vi "pco.camera_SaveMean_Example_IMAQ.vi"() -> ()   [LabVIEW 2019]
uses:
  pco.camera/Camera.lvclass
panel:
  out "rawImage":u16[][](array[numeric])
  out "Image":T1(plugin-control)
  in  "data_format":T2(ring)=enum."Mono16"
  in  "Image Index":u32 max=99
  in  "saveImages":bool
  in  "SavePath":path
  out "Recorded Images":u32
  in  "Quit":bool
  in  "roiY1":u64=2 min=2 max=1040 step=1
  in  "roiX1":u64=2 min=2 max=1392 step=1
  in  "roiY0":u64=1 min=1 max=1039 step=1
  in  "roiX0":u64=1 min=1 max=1391 step=1
  out "Image Height":u16
  out "Image Width":u16
  in  "dwImgCount":u32=10 caption="Required Number of Images" max=4023
  out "Error":errorcluster {"code" format="%x"}
  # "This example shows how to record an image sequence, get the mean of that sequence and save it to file afterwards.\nIt is a good starting point for writing own applications.\nBut it will not be fail save, i.e. doesnt react on errors, just handles them forward to the end\n\nUsage:\nSelect your required image count you want to average over before you start the program.\nOnce started, the camera class will be initialized and images will be recorded automatically.\nTWhen acquisition has finished the mean image is read and shown.\nNow you can crop the image using the ROI parameters and select a file path.\nBy clicking save, the mean image is saved with the selected file format using the current roi setting\nThis also finishes the program and will force an exit of the camera class"
  # "pco.labview"
  # "Camera Setup"
  # "Recording Control"
  # "Parameters for image readout"
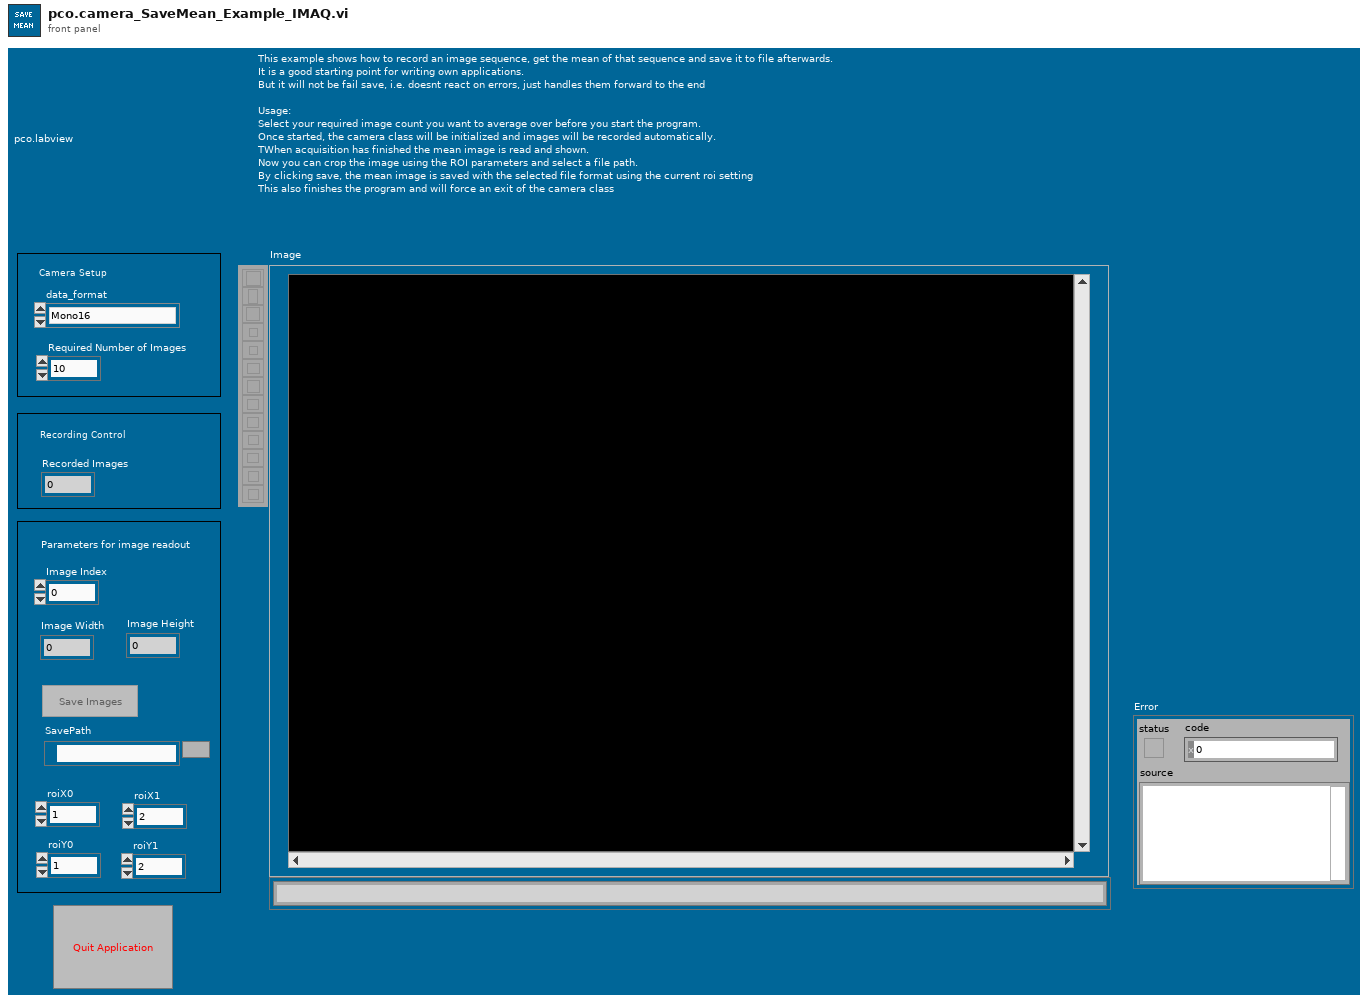
[diagram p1: front panel]
types:
  T1 = typedef "IMAQ Image.ctl" = refnum<image>
  T2 = enum16{"Undefined", "Mono8", "Mono16", "BGRA8", "RGBA8", "BGRA16", "RGBA16", "CompressedMono8"}
  T3 = enum8{"Enabled", "Disabled", "Disabled and Grayed Out"}
  T4 = enum16{"sequence", "sequence non blocking", "ring buffer", "fifo", "sequence_dpcore", "sequence_non_blocking_dpcore", "ring_buffer_dpcore", "fifo_dpcore", "tif", "multitif", "pcoraw", "b16", "dicom", "multidicom"}
  T5 = typedef "Image Type" = u32
  T6 = typedef "Camera.lvclass/binning.ctl" = cluster{"vert":u16, "horz":u16}
  T7 = cluster{"exposure_time_s":dbl, "delay_time_s":dbl, "roi":cluster{"x0":u64, "y0":u64, "x1":u64, "y1":u64}, "timestamp_mode":u16, "pixelrate":u32, "trigger_mode":u16, "acquire_mode":u16, "metadata_mode":u16, "noisefilter_mode":u16, "binning":T6}
  T8 = typedef "Color (U64)" = cluster{"Plane 3 (Blue)":u16, "Plane 2 (Green)":u16, "Plane 1 (Red)":u16, "Plane 4 (alpha)":u16}
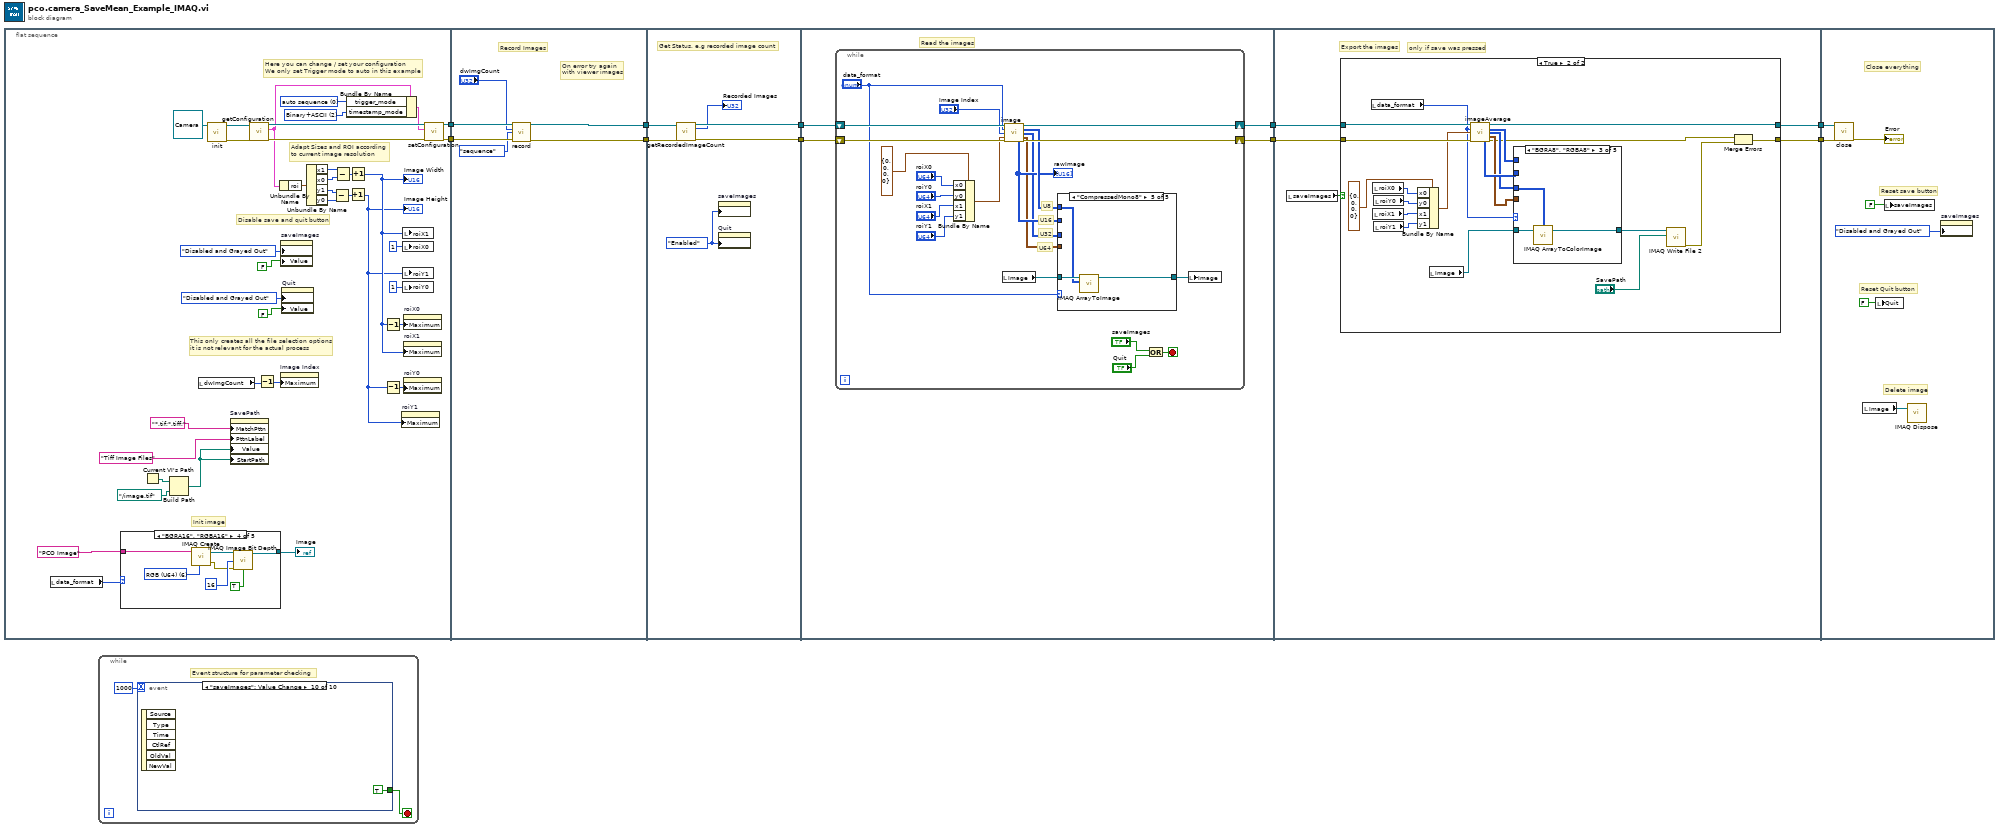
[diagram p0: block diagram]
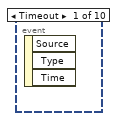
[diagram p2: hidden frame]
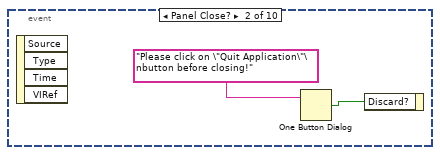
[diagram p3: hidden frame]
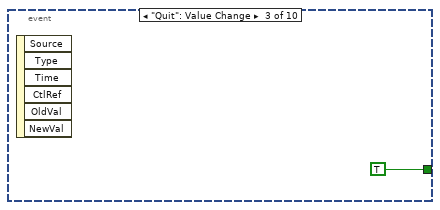
[diagram p4: hidden frame]
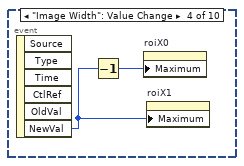
[diagram p5: hidden frame]
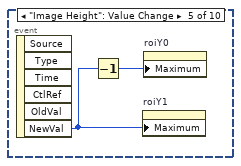
[diagram p6: hidden frame]
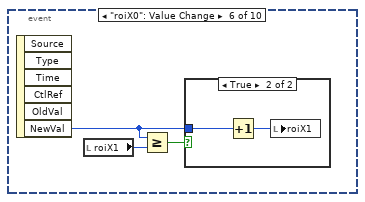
[diagram p7: hidden frame]
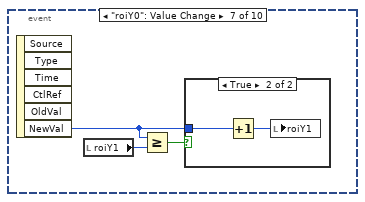
[diagram p9: hidden frame]
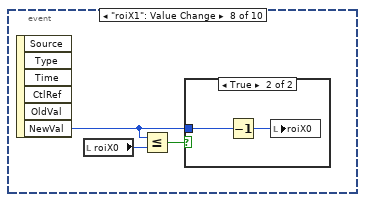
[diagram p11: hidden frame]
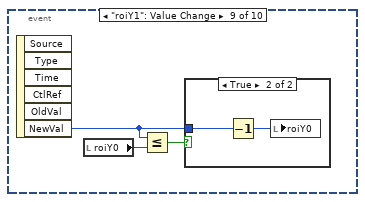
[diagram p13: hidden frame]
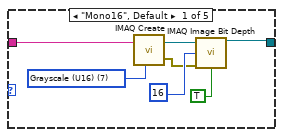
[diagram p15: hidden frame]
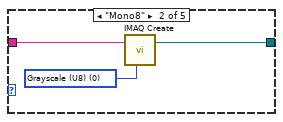
[diagram p16: hidden frame]
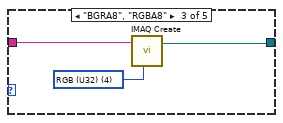
[diagram p17: hidden frame]
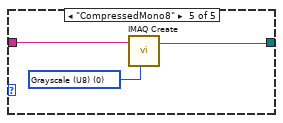
[diagram p18: hidden frame]
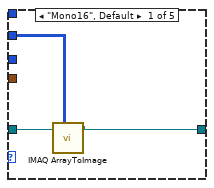
[diagram p19: hidden frame]
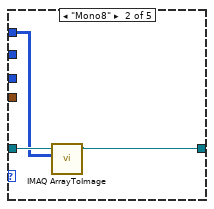
[diagram p20: hidden frame]
diagram:
  n1 = flat-sequence {
    tunnel: [w39] -> w10
    tunnel: [w38] -> w9
    tunnel: w10 -> [w77]
    tunnel: w9 -> [w76]
    tunnel: [w74] -> w8
    tunnel: [w73] -> w7
    tunnel: w8 -> [w83]
    tunnel: w7 -> [w82]
    tunnel: [w81] -> w6
    tunnel: [w80] -> w5
    tunnel: w6 -> [w86]
    tunnel: w5 -> [w87]
    tunnel: [w85] -> w4
    tunnel: [w84] -> w2
    tunnel: w4 -> [w127]
    tunnel: [w126] -> w3
    tunnel: w2 -> [w125]
    tunnel: [w124] -> w1
    tunnel: w3 -> [w172]
    tunnel: w1 -> [w171]
    frame #0 {
      w23 = u16 2 items=["OFF", "Binary", "Binary+ASCII", "ASCII"] ("TimestampMode")
      w45 = u16 0 items=["auto sequence"=0, "software trigger"=1, "external exposure start & software trigger"=2, "external exposure control"=3, "external synchronized"=4, "fast external exposure control"=5, "external CDS control"=6, "slow external exposure control"=7, "external synchronized HDSDI"=258] ("TriggerMode")
      # "Init image"
      # "This only creates all the file selection options\nit is not relevant for the actual process"
      # "Adapt Sizes and ROI according\nto current image resolution"
      # "Disable save and quit button"
      # "Here you can change / set your configuration\nWe only set Trigger mode to auto in this example"
      n2 = local read "data_format"() -> (w13:T2)
      n3 = case shown="\"BGRA16\", \"RGBA16\"" w13 {
        tunnel: "PCO Image" ("Image Name") -> [w54 w58 w60 w67 w70]
        tunnel: [w49 w56 w59 w63 w69] -> w12
        frame "Mono16", Default {
          w55 = T5 7 items=["Grayscale (U8)", "Grayscale (I16)", "Grayscale (SGL)", "Complex (CSG)", "RGB (U32)", "HSL (U32)", "RGB (U64)", "Grayscale (U16)"] ("Image Type")
          n4 = call "IMAQ Create"("Image Name"=w54, "Image Type"=w55) -> ("New Image"=w51:T1, "error out"=w50:errorcluster)  [unwired: 3 in]
          n5 = call "IMAQ Image Bit Depth"("Image"=w51, "Bit Depth (0)"=u32 16, "error in (no error)"=w50, "Get/Set Bit Depth? (Set)"=TRUE) -> ("Image Out"=w49:T1)  [unwired: 9 in, 2 out]
        }
        frame "Mono8" {
          w57 = T5 0 items=["Grayscale (U8)", "Grayscale (I16)", "Grayscale (SGL)", "Complex (CSG)", "RGB (U32)", "HSL (U32)", "RGB (U64)", "Grayscale (U16)"] ("Image Type")
          n6 = call "IMAQ Create"("Image Name"=w58, "Image Type"=w57) -> ("New Image"=w56:T1)  [unwired: 3 in, 1 out]
        }
        frame "BGRA8", "RGBA8" {
          w61 = T5 4 items=["Grayscale (U8)", "Grayscale (I16)", "Grayscale (SGL)", "Complex (CSG)", "RGB (U32)", "HSL (U32)", "RGB (U64)", "Grayscale (U16)"] ("Image Type")
          n7 = call "IMAQ Create"("Image Name"=w60, "Image Type"=w61) -> ("New Image"=w59:T1)  [unwired: 3 in, 1 out]
        }
        frame "BGRA16", "RGBA16" {
          w68 = T5 6 items=["Grayscale (U8)", "Grayscale (I16)", "Grayscale (SGL)", "Complex (CSG)", "RGB (U32)", "HSL (U32)", "RGB (U64)", "Grayscale (U16)"] ("Image Type")
          n8 = call "IMAQ Create"("Image Name"=w67, "Image Type"=w68) -> ("New Image"=w64:T1, "error out"=w62:errorcluster)  [unwired: 3 in]
          n9 = call "IMAQ Image Bit Depth"("Image"=w64, "Bit Depth (0)"=u32 16, "error in (no error)"=w62, "Get/Set Bit Depth? (Set)"=TRUE) -> ("Image Out"=w63:T1)  [unwired: 9 in, 2 out]
        }
        frame "CompressedMono8" {
          w71 = T5 0 items=["Grayscale (U8)", "Grayscale (I16)", "Grayscale (SGL)", "Complex (CSG)", "RGB (U32)", "HSL (U32)", "RGB (U64)", "Grayscale (U16)"] ("Image Type")
          n10 = call "IMAQ Create"("Image Name"=w70, "Image Type"=w71) -> ("New Image"=w69:T1)  [unwired: 3 in, 1 out]
        }
      }
      "Image" <- w12
      n11 = Current VI's Path() -> (path=w20:path)
      n12 = Build Path(base path=w20, name or relative path=path "../image.tif" ("SavePath")) -> (appended path=w17:path)
      n13 = local read "dwImgCount"() -> (w15:u32)
      n14 = call-dynamic "init.vi"("Camera in"=refnum<class "Camera.lvclass"> refnum ("PCOCamera in")) -> ("Camera out"=w47:refnum<class "Camera.lvclass">, "error out"=w46:errorcluster)  [unwired: 8 in]
      n15 = property on="SavePath" class="Path"("MatchPttn"="*.tif;*.tiff;" ("pattern (all files)"), "PttnLabel"="Tiff Image Files" ("pattern label"), "Value"=w17, "StartPath"=w17) -> ()  [unwired: 2 in, 2 out]
      n16 = call-dynamic "getConfiguration.vi"("error in (no error)"=w46, "Camera in"=w47) -> ("error out"=w43:errorcluster, "configuration"=w33:T7, "Camera out"=w44:refnum<class "Camera.lvclass">)  [unwired: 7 in]
      n17 = Decrement(x=w15) -> (x-1=w16:u32)
      n18 = Unbundle By Name(w33) -> ("roi"=w32:cluster{"x0":u64, "y0":u64, "x1":u64, "y1":u64})
      n19 = property on="Image Index" class="DigNum (strict)"("Maximum"=w16) -> ()  [unwired: 2 in, 2 out]
      n20 = property on="saveImages" class="Bool (strict)"("DisabledEnum"=T3."Disabled and Grayed Out" ("Disabled"), "Value"=FALSE ("Stop")) -> ()  [unwired: 2 in, 2 out]
      n21 = property on="Quit" class="Bool (strict)"("DisabledEnum"=T3."Disabled and Grayed Out" ("Disabled"), "Value"=FALSE ("Stop")) -> ()  [unwired: 2 in, 2 out]
      n22 = Unbundle By Name(w32) -> ("x1"=w30:u64, "x0"=w31:u64, "y1"=w28:u64, "y0"=w29:u64)
      n23 = Subtract(x=w28, y=w29) -> (x-y=w26:u64)
      n24 = Subtract(x=w30, y=w31) -> (x-y=w27:u64)
      n25 = Bundle By Name(cluster=w33, "trigger_mode"=w45, "timestamp_mode"=w23) -> (w42:T7)
      n26 = Increment(x=w26) -> (x+1=w24:u64)
      "Image Height" <- w24
      n27 = Increment(x=w27) -> (x+1=w25:u64)
      "Image Width" <- w25
      n28 = Decrement(x=w25) -> (x-1=w35:u64)
      n29 = Decrement(x=w24) -> (x-1=w34:u64)
      n30 = property on="roiY1" class="DigNum (strict)"("Maximum"=w24) -> ()  [unwired: 2 in, 2 out]
      n31 = local write "roiX1"(w25) -> ()
      n32 = local write "roiX0"(u16 1 ("roiY0")) -> ()
      n33 = local write "roiY1"(w24) -> ()
      n34 = local write "roiY0"(u16 1 ("roiY0")) -> ()
      n35 = property on="roiX0" class="DigNum (strict)"("Maximum"=w35) -> ()  [unwired: 2 in, 2 out]
      n36 = property on="roiX1" class="DigNum (strict)"("Maximum"=w25) -> ()  [unwired: 2 in, 2 out]
      n37 = property on="roiY0" class="DigNum (strict)"("Maximum"=w34) -> ()  [unwired: 2 in, 2 out]
      n38 = call-dynamic "setConfiguration.vi"("error in (no error)"=w43, "configuration"=w42, "Camera in"=w44) -> ("error out"=w38:errorcluster, "Camera out"=w39:refnum<class "Camera.lvclass">)  [unwired: 7 in]
    }
    frame #1 {
      # "On error try again \nwith viewer images"
      # "Record Images"
      n39 = call-dynamic "record.vi"("Camera in"=w77, "num_images"="dwImgCount", "record_mode"=T4."sequence", "error in (no error)"=w76) -> ("Camera out"=w74:refnum<class "Camera.lvclass">, "error out"=w73:errorcluster)  [unwired: 10 in]
    }
    frame #2 {
      w78 = T3."Enabled" ("Disabled")
      # "Get Status, e.g recorded image count"
      n40 = call-dynamic "getRecordedImageCount.vi"("Camera in"=w83, "error in (no error)"=w82) -> ("Camera out"=w81:refnum<class "Camera.lvclass">, "recorded_image_count"=→"Recorded Images":u32, "error out"=w80:errorcluster)  [unwired: 11 in]
      n41 = property on="saveImages" class="Bool (strict)"("DisabledEnum"=w78) -> ()  [unwired: 2 in, 2 out]
      n42 = property on="Quit" class="Bool (strict)"("DisabledEnum"=w78) -> ()  [unwired: 2 in, 2 out]
    }
    frame #3 {
      # "Read the images"
      n43 = while {
        shift-right: [w106] -> w85
        shift-left: w86 -> [w108]
        shift-right: [w101] -> w84
        shift-left: w87 -> [w107]
        stop <- w99 stop-if-true
        # "U64"
        # "U32"
        # "U16"
        # "U8"
        n44 = Bundle By Name(cluster=cluster{"x0":u64, "y0":u64, "x1":u64, "y1":u64} {"x0"=0, "y0"=0, "x1"=0, "y1"=0} ("roi"), "x0"="roiX0", "y0"="roiY0", "x1"="roiX1", "y1"="roiY1") -> (w97:cluster{"x0":u64, "y0":u64, "x1":u64, "y1":u64})
        n45 = local read "Image"() -> (w90:T1)
        n46 = call-dynamic "image.vi"("Camera in"=w108, "data_format"="data_format", "image_index"="Image Index", "roi"=w97, "error in (no error)"=w107) -> ("Camera out"=w106:refnum<class "Camera.lvclass">, "image (U8)"=w94:u8[][], "image (U32)"=w92:u32[][], "image (U64)"=w91:T8[][], "raw_image (U16)"=w93:u16[][], "error out"=w101:errorcluster)  [unwired: 3 in, 2 out]
        "rawImage" <- w93
        n47 = case shown="\"CompressedMono8\"" "data_format" {
          tunnel: w90 -> [w111 w114 w117 w120 w123]
          tunnel: [w109 w112 w116 w118 w122] -> w89
          tunnel: w91 -> [_ _ _ w119 _]
          tunnel: w92 -> [_ _ w115 _ _]
          tunnel: w94 -> [_ w113 _ _ w121]
          tunnel: w93 -> [w110 _ _ _ _]
          frame "Mono16", Default {
            n48 = call "IMAQ ArrayToImage"("Image Pixels (U16)"=w110, "Image"=w111) -> ("Image Out"=w109:T1)  [unwired: 8 in, 1 out]
          }
          frame "Mono8" {
            n49 = call "IMAQ ArrayToImage"("Image Pixels (U8)"=w113, "Image"=w114) -> ("Image Out"=w112:T1)  [unwired: 8 in, 1 out]
          }
          frame "BGRA8", "RGBA8" {
            n50 = call "IMAQ ArrayToColorImage"("Image Pixels (U32)"=w115, "Image"=w117) -> ("Image Out"=w116:T1)  [unwired: 3 in, 1 out]
          }
          frame "BGRA16", "RGBA16" {
            n51 = call "IMAQ ArrayToColorImage"("Image"=w120, "Image Pixels (U64)"=w119) -> ("Image Out"=w118:T1)  [unwired: 3 in, 1 out]
          }
          frame "CompressedMono8" {
            n52 = call "IMAQ ArrayToImage"("Image Pixels (U8)"=w121, "Image"=w123) -> ("Image Out"=w122:T1)  [unwired: 8 in, 1 out]
          }
        }
        n53 = Or(x="saveImages", y="Quit") -> (x .or. y?=w99:bool)
        n54 = local write "Image"(w89) -> ()
      }
    }
    frame #4 {
      # "only if save was pressed"
      # "Export the images"
      n55 = local read "saveImages"() -> (w128:bool)
      n56 = case shown="True" w128 {
        tunnel: w127 -> [w130 w149]
        tunnel: [w130 w138] -> w126
        tunnel: w125 -> [w129 w150]
        tunnel: [w129 w136] -> w124
        frame False {
        }
        frame True {
          n57 = local read "data_format"() -> (w134:T2)
          n58 = local read "roiX0"() -> (w147:u64)
          n59 = local read "roiX1"() -> (w145:u64)
          n60 = local read "roiY0"() -> (w146:u64)
          n61 = local read "roiY1"() -> (w144:u64)
          n62 = Bundle By Name(cluster=cluster{"x0":u64, "y0":u64, "x1":u64, "y1":u64} {"x0"=0, "y0"=0, "x1"=0, "y1"=0} ("roi"), "x0"=w147, "y0"=w146, "x1"=w145, "y1"=w144) -> (w143:cluster{"x0":u64, "y0":u64, "x1":u64, "y1":u64})
          n63 = local read "Image"() -> (w135:T1)
          n64 = call-dynamic "imageAverage.vi"("Camera in"=w149, "data_format"=w134, "roi"=w143, "error in (no error)"=w150) -> ("Camera out"=w138:refnum<class "Camera.lvclass">, "image (U8)"=w142:u8[][], "image (U32)"=w140:u32[][], "image (U64)"=w139:T8[][], "raw_image (U16)"=w141:u16[][], "error out"=w137:errorcluster)  [unwired: 6 in]
          n65 = case shown="\"BGRA8\", \"RGBA8\"" w134 {
            tunnel: w135 -> [w153 w156 w159 w162 w165]
            tunnel: [w151 w154 w158 w160 w164] -> w132
            tunnel: w139 -> [_ _ _ w161 _]
            tunnel: w140 -> [_ _ w157 _ _]
            tunnel: w142 -> [_ w155 _ _ w163]
            tunnel: w141 -> [w152 _ _ _ _]
            frame "Mono16", Default {
              n66 = call "IMAQ ArrayToImage"("Image Pixels (U16)"=w152, "Image"=w153) -> ("Image Out"=w151:T1)  [unwired: 8 in, 1 out]
            }
            frame "Mono8" {
              n67 = call "IMAQ ArrayToImage"("Image Pixels (U8)"=w155, "Image"=w156) -> ("Image Out"=w154:T1)  [unwired: 8 in, 1 out]
            }
            frame "BGRA8", "RGBA8" {
              n68 = call "IMAQ ArrayToColorImage"("Image Pixels (U32)"=w157, "Image"=w159) -> ("Image Out"=w158:T1)  [unwired: 3 in, 1 out]
            }
            frame "BGRA16", "RGBA16" {
              n69 = call "IMAQ ArrayToColorImage"("Image"=w162, "Image Pixels (U64)"=w161) -> ("Image Out"=w160:T1)  [unwired: 3 in, 1 out]
            }
            frame "CompressedMono8" {
              n70 = call "IMAQ ArrayToImage"("Image Pixels (U8)"=w163, "Image"=w165) -> ("Image Out"=w164:T1)  [unwired: 8 in, 1 out]
            }
          }
          n71 = call-poly "IMAQ Write File 2"("File Path"="SavePath", "Image"=w132) -> ("error out"=w133:errorcluster)  [unwired: 8 in, 1 out]
          n72 = Merge Errors(w137, w133) -> (w136:errorcluster)
        }
      }
    }
    frame #5 {
      # "Delete image"
      # "Reset Quit button"
      # "Close everything"
      # "Reset save button"
      n73 = call-dynamic "close.vi"("error in (no error)"=w171, "Camera in"=w172) -> ("error out"=→"Error":errorcluster)  [unwired: 9 in]
      n74 = local read "Image"() -> (w166:T1)
      n75 = local write "Quit"(FALSE ("Stop")) -> ()
      n76 = local write "saveImages"(FALSE ("Stop")) -> ()
      n77 = call "IMAQ Dispose"("Image"=w166) -> ()  [unwired: 5 in, 1 out]
      n78 = property on="saveImages" class="Bool (strict)"("DisabledEnum"=T3."Disabled and Grayed Out" ("Disabled")) -> ()  [unwired: 2 in, 2 out]
    }
  }
  n79 = while {
    stop <- w173 stop-if-true
    # "Event structure for parameter checking"
    n80 = event shown="[9] \"saveImages\": Value Change" {
      selector: _ -> [_ _ _ _ _ _ _ _ _ _]
      dyn-events: _ -> [_ _ _ _ _ _ _ _ _ _]
      timeout: 1000 -> [_ _ _ _ _ _ _ _ _ _]
      tunnel: [_ _ TRUE _ _ _ _ _ _ TRUE] -> w173
      event Timeout {
        n81 = event-data() -> ()  [unwired: 1 in, 3 out]
      }
      event Panel Close? {
        n82 = event-data() -> ()  [unwired: 1 in, 4 out]
        n83 = One Button Dialog(message="Please click on \"Quit Application\"\nbutton before closing!") -> (true=w175:bool)  [unwired: 1 in]
        n84 = event-data("Discard?"=w175) -> ()  [unwired: 1 in, 1 out]
      }
      event "Quit": Value Change {
        n85 = event-data() -> ()  [unwired: 1 in, 6 out]
      }
      event "Image Width": Value Change {
        n86 = event-data() -> ("NewVal"=w178:u16)  [unwired: 1 in, 5 out]
        n87 = Decrement(x=w178) -> (x-1=w179:u16)
        n88 = property on="roiX0" class="DigNum (strict)"("Maximum"=w179) -> ()  [unwired: 2 in, 2 out]
        n89 = property on="roiX1" class="DigNum (strict)"("Maximum"=w178) -> ()  [unwired: 2 in, 2 out]
      }
      event "Image Height": Value Change {
        n90 = event-data() -> ("NewVal"=w180:u16)  [unwired: 1 in, 5 out]
        n91 = Decrement(x=w180) -> (x-1=w181:u16)
        n92 = property on="roiY1" class="DigNum (strict)"("Maximum"=w180) -> ()  [unwired: 2 in, 2 out]
        n93 = property on="roiY0" class="DigNum (strict)"("Maximum"=w181) -> ()  [unwired: 2 in, 2 out]
      }
      event "roiX0": Value Change {
        n94 = event-data() -> ("NewVal"=w182:u64)  [unwired: 1 in, 5 out]
        n95 = local read "roiX1"() -> (w184:u64)
        n96 = Greater Or Equal?(x=w182, y=w184) -> (x >= y?=w183:bool)
        n97 = case shown="True" w183 {
          tunnel: w182 -> [_ w186]
          frame False {
          }
          frame True {
            n98 = Increment(x=w186) -> (x+1=w185:u64)
            n99 = local write "roiX1"(w185) -> ()
          }
        }
      }
      event "roiY0": Value Change {
        n100 = event-data() -> ("NewVal"=w187:u64)  [unwired: 1 in, 5 out]
        n101 = local read "roiY1"() -> (w189:u64)
        n102 = Greater Or Equal?(x=w187, y=w189) -> (x >= y?=w188:bool)
        n103 = case shown="True" w188 {
          tunnel: w187 -> [_ w191]
          frame False {
          }
          frame True {
            n104 = Increment(x=w191) -> (x+1=w190:u64)
            n105 = local write "roiY1"(w190) -> ()
          }
        }
      }
      event "roiX1": Value Change {
        n106 = event-data() -> ("NewVal"=w192:u64)  [unwired: 1 in, 5 out]
        n107 = local read "roiX0"() -> (w194:u64)
        n108 = Less Or Equal?(x=w192, y=w194) -> (x <= y?=w193:bool)
        n109 = case shown="True" w193 {
          tunnel: w192 -> [_ w196]
          frame False {
          }
          frame True {
            n110 = Decrement(x=w196) -> (x-1=w195:u64)
            n111 = local write "roiX0"(w195) -> ()
          }
        }
      }
      event "roiY1": Value Change {
        n112 = event-data() -> ("NewVal"=w197:u64)  [unwired: 1 in, 5 out]
        n113 = local read "roiY0"() -> (w199:u64)
        n114 = Less Or Equal?(x=w197, y=w199) -> (x <= y?=w198:bool)
        n115 = case shown="True" w198 {
          tunnel: w197 -> [_ w201]
          frame False {
          }
          frame True {
            n116 = Decrement(x=w201) -> (x-1=w200:u64)
            n117 = local write "roiY0"(w200) -> ()
          }
        }
      }
      event "saveImages": Value Change {
        n118 = event-data() -> ()  [unwired: 1 in, 6 out]
      }
    }
  }
